vi "TTA_Pause.vi"(8 "error in":errorcluster, 11 "Pause (ms)":u32) -> (0 "error out":errorcluster)   [LabVIEW 2016]
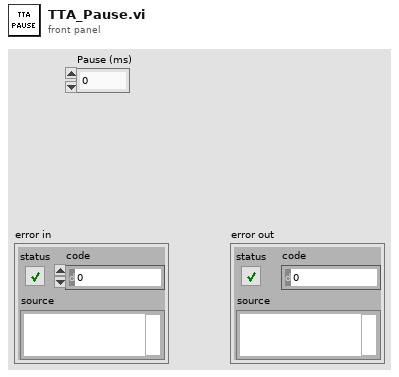
[diagram p1: front panel]
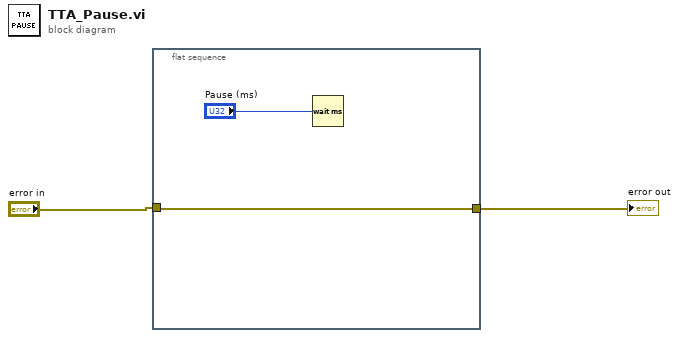
[diagram p0: block diagram]
diagram:
  n1 = flat-sequence {
    tunnel: "error in" -> [w4]
    tunnel: [w4] -> w1
    frame #0 {
      n2 = Wait (ms)(milliseconds to wait="Pause (ms)") -> ()  [unwired: 1 out]
    }
  }
  "error out" <- w1
